vi "Do Request.vi"(7 "Processing In":refnum<class "Processing.lvclass">, 11 "AudioSummaryController in":refnum<class "AudioSummaryController.lvclass">) -> (0 "error out":errorcluster, 5 "Processing":refnum<class "Processing.lvclass">)   [LabVIEW 2022 SP3, in "VMR Server.lvlib" / "AudioSummaryController.lvclass"]
doc: "A controller's main job is to respond to a request by generating a response. The response value must be specified by calling Set Response.vi on the Processing class that's passed through the VI otherwise an error will be generated.\n\nThere are several helpers available for common response types:\nGenerating HTML content programmatically - Create Basic Response.vi\nStreaming a file from disk - Create File Response.vi\nRedirecting the user to another URL - Create Redirect Response.vi\n\nFile responses are streamed in chunks and do not load the entire file into memory at once to send in the response which allows serving large files more efficiently."
uses:
  AudioSummaryController.lvclass
  <vilib>/IlluminatedG/IG HTTP Server/HTTP Server/Processing/Processing.lvclass
  AudioSummaryController.lvclass/AudioSummaryController.ctl
  VMR Actor API/VMR Actor API.lvclass
  <vilib>/IlluminatedG/IG HTTP Utils/HTTP Utils/Response/Response.lvclass
  C:/dev/lv/2022/touchcontrol/VMR Server/VMR Actor API/VMR Actor API.lvclass
  C:/Program Files (x86)/National Instruments/LabVIEW 2022/vi.lib/IlluminatedG/IG HTTP Server/HTTP Server/Service/Service.lvclass
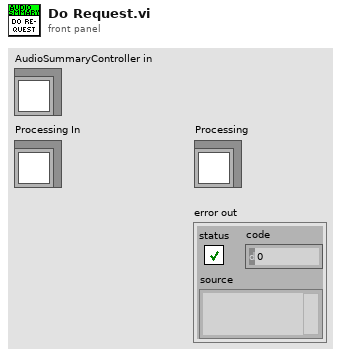
[diagram p1: front panel]
types:
  T1 = typedef "VMR Server Shared.lvlib/Audio Summary.ctl" = cluster{"Route":bool[][], "Channels":T2[]}
  T2 = typedef "VMR Server Shared.lvlib/Channel.ctl" = cluster{"Gain":dbl, "Muted":bool, "Levels":cluster{"L":dbl, "R":dbl}}
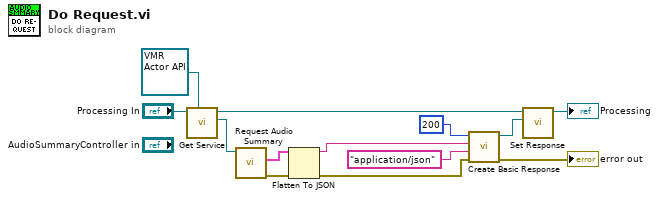
[diagram p0: block diagram]
diagram:
  n1 = call <vilib>:"Get Service.vi"("Service Type"=refnum<class "VMR Actor API.lvclass"> refnum ("VMR Server.lvlib:VMR Actor API.lvclass"), "Processing in"="Processing In") -> ("Service"=w11:refnum<class "VMR Actor API.lvclass">, "Processing out"=w5:refnum<class "Processing.lvclass">)  [unwired: 7 in, 1 out]
  n2 = call "Request Audio Summary.vi"("VMR Actor API in"=w11) -> ("error out"=w2:errorcluster, "Audio Summary"=w10:T1)  [unwired: 9 in]
  n3 = Flatten To JSON(anything=w10, error in (no error)=w2) -> (JSON string=w8:string, 11:w1:errorcluster)  [unwired: 1 in]
  n4 = call <vilib>:"Create Basic Response.vi"("error in (no error)"=w1, "Content-Type (text/plain)"="application/json", "Payload"=w8, "Status Code"=u16 200) -> ("error out"=→"error out":errorcluster, "Response out"=w4:refnum<class "Response.lvclass">)  [unwired: 6 in]
  n5 = call <vilib>:"Set Response.vi"("Response"=w4, "Processing in"=w5) -> ("Processing out"=→"Processing":refnum<class "Processing.lvclass">)  [unwired: 9 in]
